vi "公式写入.vi"(7 "公式":cluster{"X^2":dbl, "X":dbl, "b":dbl}, 8 "error in (no error)":errorcluster caption="错误输入（无错误）", 9 "量程":enum16{"低量程", "高量程"}(ring), 10 "测量模式":T1(ring), 11 "测量参数":u16(ring) items=["总磷"=1, "总氮"=2, "氨氮"=3, "COD"=22]) -> (0 "error out":errorcluster caption="错误输出")   [LabVIEW 2016, in "斯坦道总磷.lvlib"]
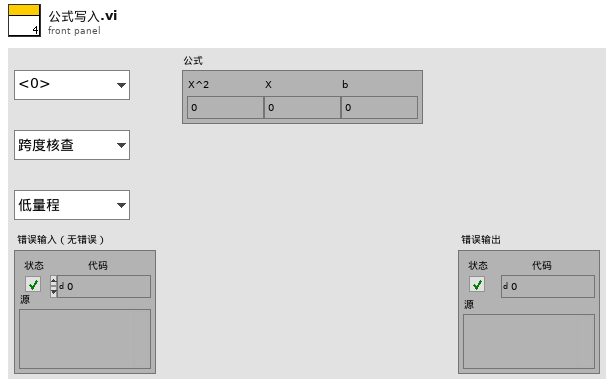
[diagram p1: front panel]
types:
  T1 = enum16{"跨度核查", "水样测量", "零点核查", "标样核查", "加标回收", "快捷测试", "空白校准", "标样校准"}
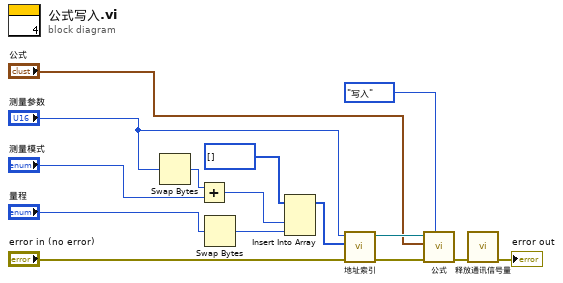
[diagram p0: block diagram]
diagram:
  n1 = Swap Bytes(anything="测量参数") -> (byte swapped=w13:u16)
  n2 = Add(x=w13, y="测量模式") -> (x+y=w15:u16)
  n3 = Swap Bytes(anything="量程") -> (byte swapped=w11:u16)
  n4 = Insert Into Array(array=u16[] [] ("数组"), new element #1=w15, new element #2=w11) -> (w4:u16[])  [unwired: 1 in]
  n5 = call "地址索引.vi"("error in (no error)"="error in (no error)", "values"=w4, "测量参数"="测量参数") -> ("error out"=w8:errorcluster, "MB session out"=w9:refnum<class "MB_Master.lvclass">)  [unwired: 7 in]
  n6 = call "公式.vi"("功能"=enum16{"读取", "写入"}."写入", "error in (no error)"=w8, "公式写入"="公式", "MB session in"=w9) -> ("error out"=w6:errorcluster)  [unwired: 5 in, 2 out]
  n7 = call "释放通讯信号量.vi"("error in (no error)"=w6) -> ("error out"=→"error out":errorcluster)  [unwired: 10 in]
